vi "TimeInterpRotation2d_SetMaxTime.vi"(9 "Max Time":dbl, 11 "in TimeInterpRotation":T1 {"RotationValues"."SIN" format="%13.4f"; "RotationValues"."COS" format="%13.4f"; "RotationValues"."VALUE" format="%13.4f"}) -> (3 "out TimeInterpRotation":T1 {"RotationValues"."SIN" format="%13.4f"; "RotationValues"."COS" format="%13.4f"; "RotationValues"."VALUE" format="%13.4f"})   [LabVIEW 2019, in "Trajectory_Library.lvlib"]
doc: "Sets the maximum time period that should be stored in the buffer.\n\nInputs:\n - In TimeInterpRotation2d -- Input data cluster.\n - Max Time -- Maximum time period to store in the buffer (seconds)\n\nOutputs:\n - Out TimeInterpRotation2d -- Updated data cluster."
uses:
  Trajectory_Library.lvlib
  TypeDef/TIME_INTERPOLATABLE_ROTATION2D.ctl
  TypeDef/ROTATION2D.ctl
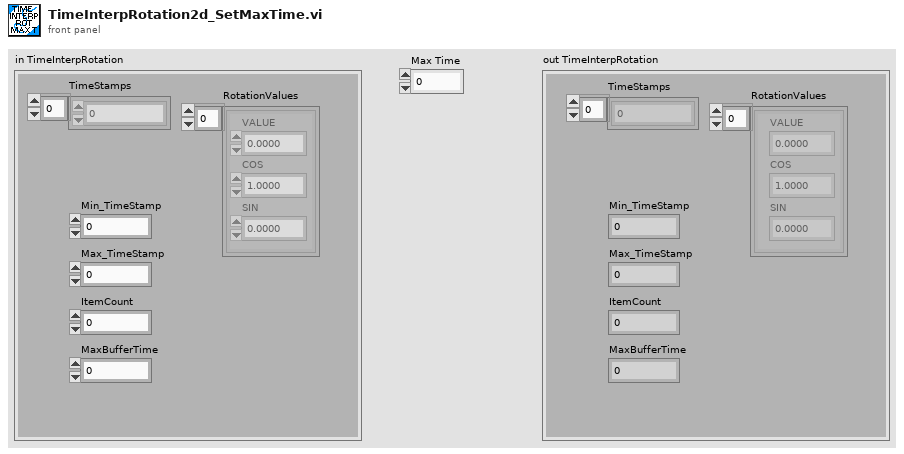
[diagram p1: front panel]
types:
  T1 = typedef "Trajectory_Library.lvlib/TIME_INTERPOLATABLE_ROTATION2D.ctl" = cluster{"TimeStamps":dbl[], "RotationValues":T2[], "Min_TimeStamp":dbl, "Max_TimeStamp":dbl, "ItemCount":i32, "MaxBufferTime":dbl}
  T2 = typedef "Trajectory_Library.lvlib/ROTATION2D.ctl" = cluster{"VALUE":dbl, "COS":dbl, "SIN":dbl}
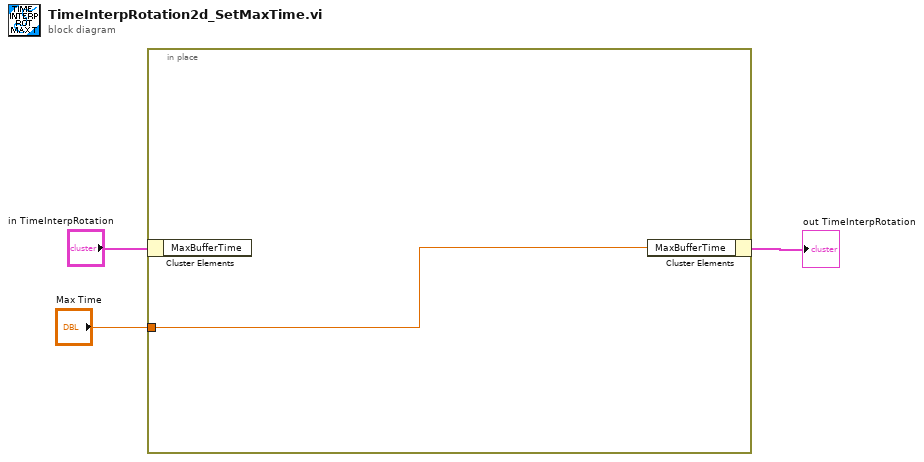
[diagram p0: block diagram]
diagram:
  n1 = in-place {
    in-place-border: "Max Time" -> [w4]
    n2 = in-place-cluster #1("in TimeInterpRotation") -> ()  [unwired: 1 out]
    n3 = in-place-cluster #1("MaxBufferTime"=w4) -> (→"out TimeInterpRotation":T1)
  }
